vi "PD3_model_calc.vi"(7 "mode":bool, 11 "pos_in":dbl[](array[numeric])=[262.0, 120.4]) -> (2 "-I_out":dbl, 3 "+I_out":dbl)   [LabVIEW 2024]
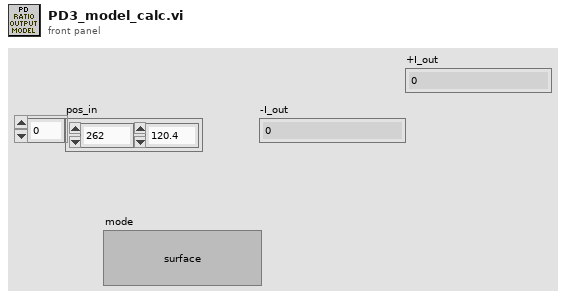
[diagram p1: front panel]
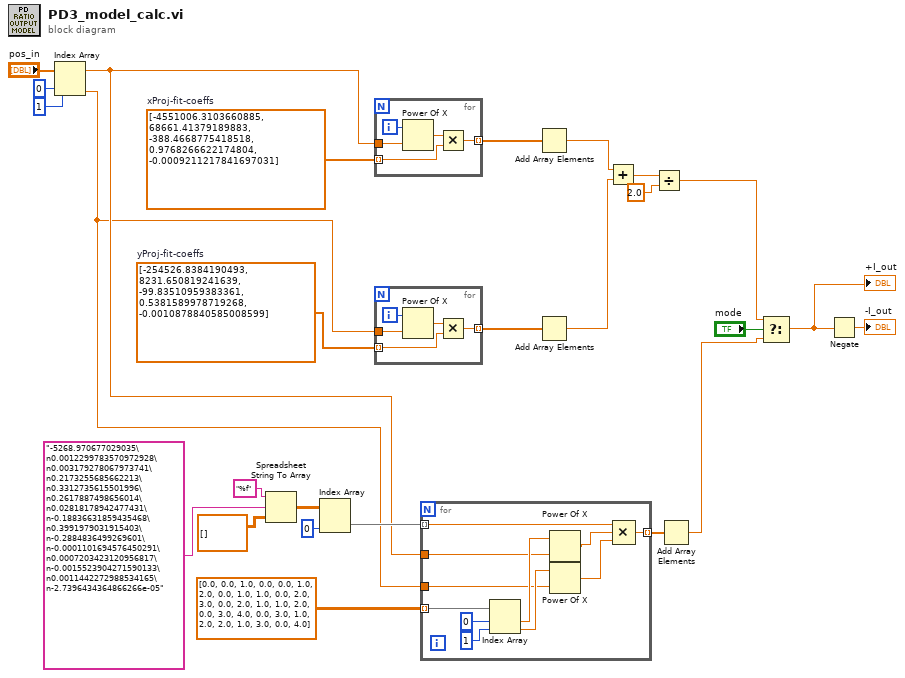
[diagram p0: block diagram]
diagram:
  w23 = dbl[] [-254526.8384190493, 8231.650819241639, -99.83510959383361, 0.5381589978719268, -0.0010878840585008599]  # yProj-fit-coeffs
  w25 = dbl[] [-4551006.3103660885, 68661.41379189883, -388.4668775418518, 0.9768266622174804, -0.0009211217841697031]  # xProj-fit-coeffs
  n1 = Index Array(array="pos_in", index #1=0 ("index"), index #2=1 ("index")) -> (element #1=w6:dbl, element #2=w5:dbl)
  n2 = Spreadsheet String To Array(format string="%f", spreadsheet string="-5268.970677029035\n0.0012299783570972928\n0.003179278067973741\n0.2173255685662213\n0.3312735615501996\n0.2617887498656014\n0.02818178942477431\n-0.18836631859435468\n0.3991979031915403\n-0.2884836499269601\n-0.0001101694576450291\n0.0007203423120956817\n-0.0015523904271590133\n0.0011442272988534165\n-2.7396434364866266e-05", array type (2D Dbl)=dbl[][] []) -> (array=w11:dbl[][])  [unwired: 1 in]
  n3 = Index Array(array=w11, index (col)=0 ("disabled index (col)")) -> (element=w9:dbl[])  [unwired: 1 in]
  n4 = for {
    tunnel: w6 -> [w31]
    tunnel: w25 -> [w28] mode=indexing
    tunnel: [w27] -> w26 mode=indexing
    i -> [w30]
    n5 = Power Of X(1:w31, 2:w30) -> (0:w29:dbl)
    n6 = Multiply(x=w29, y=w28) -> (x*y=w27:dbl)
  }
  n7 = for {
    tunnel: w5 -> [w36]
    tunnel: w23 -> [w33] mode=indexing
    tunnel: [w32] -> w24 mode=indexing
    i -> [w35]
    n8 = Power Of X(1:w36, 2:w35) -> (0:w34:dbl)
    n9 = Multiply(x=w34, y=w33) -> (x*y=w32:dbl)
  }
  n10 = for {
    tunnel: w9 -> [w39] mode=indexing
    tunnel: dbl[][] [[0.0, 0.0], [1.0, 0.0], [0.0, 1.0], [2.0, 0.0], [1.0, 1.0], [0.0, 2.0], [3.0, 0.0], [2.0, 1.0], [1.0, 2.0], [0.0, 3.0], [4.0, 0.0], [3.0, 1.0], [2.0, 2.0], [1.0, 3.0], [0.0, 4.0]] -> [w47] mode=indexing
    tunnel: w6 -> [w42]
    tunnel: w5 -> [w41]
    tunnel: [w40] -> w7 mode=indexing
    n11 = Index Array(array=w47, index #1=0 ("index"), index #2=1 ("index")) -> (element #1=w44:dbl, element #2=w43:dbl)
    n12 = Power Of X(1:w42, 2:w44) -> (0:w38:dbl)
    n13 = Power Of X(1:w41, 2:w43) -> (0:w37:dbl)
    n14 = Compound Arithmetic op=MULTIPLY(w39, w38, w37) -> (w40:dbl)
  }
  n15 = Add Array Elements(numeric array=w26) -> (sum=w22:dbl)
  n16 = Add Array Elements(numeric array=w24) -> (sum=w21:dbl)
  n17 = Add(x=w22, y=w21) -> (x+y=w20:dbl)
  n18 = Divide(x=w20, y=2.0) -> (x/y=w2:dbl)
  n19 = Add Array Elements(numeric array=w7) -> (sum=w3:dbl)
  n20 = Select(t=w2, s="mode", f=w3) -> (s? t:f=w1:dbl)
  "+I_out" <- w1
  n21 = Negate(x=w1) -> (-x=→"-I_out":dbl)
